vi "Start FTE Command.vi"(8 "error in":errorcluster, 10 "Start FTE":i64, 11 "CIFCorePlugin in":refnum<class "CIFCorePlugin.lvclass">) -> (0 "error out":errorcluster, 3 "CIFCorePlugin out":refnum<class "CIFCorePlugin.lvclass">)   [LabVIEW 2021, in "CIFCorePlugin.lvclass"]
uses:
  CIFCorePlugin.lvclass
  CIFCorePlugin.lvclass/CIFCorePlugin.ctl
  Typedef/gRPC to Main Command Payload.ctl
  Typedef/gRPC to Main Commands.ctl
  50968075-8c01-466c-b517-9351d77275d7.vi
  <vilib>/CIF Foundation/CIF CIPC/SubVIs/Check Error.vi
  <vilib>/CIF Foundation/CIF CIPC/SubVIs/Notify Of New Write.vi
  <vilib>/CIF Foundation/CIF CIPC/SubVIs/Get dll Path.vi
  <vilib>/CIF Foundation/CIF CIPC/SubVIs/Get Element Write Position.vi
  <vilib>/CIF Foundation/CIF CIPC/SubVIs/Get Element Info Variant.vi
  <vilib>/Utility/error.llb/Trim Whitespace.vi
  <vilib>/Utility/error.llb/Error Cluster From Error Code.vi
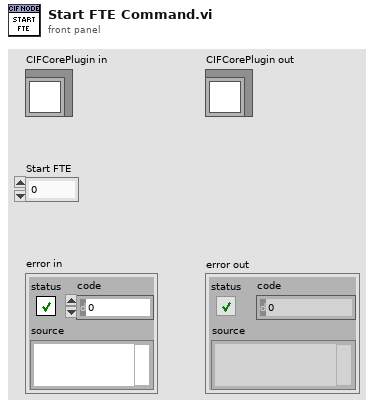
[diagram p1: front panel]
types:
  T1 = typedef "CIFCorePlugin.lvclass/gRPC to Main Command Payload.ctl" = cluster{"OOB_Rx Command":T2, "Array Index":i32}
  T2 = typedef "CIFCorePlugin.lvclass/gRPC to Main Commands.ctl" = enum8{"Start", "Pause", "Stop", "RefreshStats", "UpdateConfig", "Update Clock Map", "Connect Channel", "Force Channel", "Add Publisher Instance", "Remove Publisher Instance", "Prepare"}
  T3 = typedef "CIFCorePlugin.lvclass/gRPC to Main DVR.ctl" = refnum<data-value>
  T4 = typedef "CIFCoreCommon.lvlib/gRPC to Main Data.ctl" = cluster{"Config Data":variant, "Connections":T5[], "Forces":T6[], "Clock Conversion":T7, "Publisher Instance":T9, "Start FTE":i64}
  T5 = typedef "CIFCoreCommon.lvlib/Channel Connection Data.ctl" = cluster{"Publisher Name":string, "Subscriber Name":string, "Connection Data":u8[]}
  T6 = typedef "CIFCoreCommon.lvlib/Channel Force Data.ctl" = cluster{"Channel Name":string, "Force Data":u8[], "Force Active":bool}
  T7 = typedef "Time_CIF_U.lvlib/Clock Conversion Map.ctl" = map{u8, cluster{"Last Reset":i64, "Offset Pair":T8, "Slope":dbl, "1/Slope":dbl}}
  T8 = typedef "Time_CIF_U.lvlib/Timestamp Pair.ctl" = cluster{"System Time":i64, "External Time":i64}
  T9 = typedef "CIFCoreCommon.lvlib/FIFO Publisher.ctl" = cluster{"Publisher Name":string, "New FIFO Instance Config":T10}
  T10 = typedef "ChannelCommon.lvlib/New FIFO Instance Configuration.ctl" = cluster{"Backpressure":bool, "Bytes/Message Override":u32, "Messages/FIFO Override":u32, "Custom Data":u8[]}
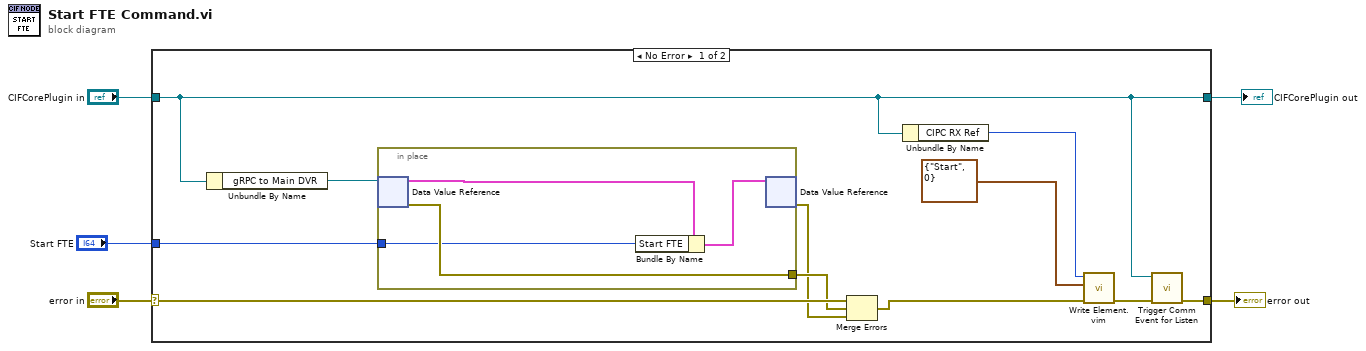
[diagram p0: block diagram]
diagram:
  n1 = case shown="No Error" "error in" {
    selector: "error in" -> [w14 w22]
    tunnel: [w7 w22] -> w2
    tunnel: "CIFCorePlugin in" -> [w6 w21]
    tunnel: [w6 w21] -> w3
    tunnel: "Start FTE" -> [w10 _]
    frame No Error {
      n2 = Unbundle By Name(w6) -> ("gRPC to Main DVR"=w15:T3)
      n3 = in-place {
        in-place-border: w10 -> [w17]
        in-place-border: [w19] -> w13
        n4 = in-place-dvr #1(w15) -> (w18:T4, w19:errorcluster)
        n5 = Bundle By Name(cluster=w18, "Start FTE"=w17) -> (w20:T4)
        n6 = in-place-dvr #1(w20) -> (w12:errorcluster)  [unwired: 1 out]
      }
      n7 = Merge Errors(w14, w13, w12) -> (w11:errorcluster)
      n8 = Unbundle By Name(w6) -> ("CIPC RX Ref"=w16:u64)
      n9 = call "Write Element.vim"("error in (no error)"=w11, "Data in"=T1 {"OOB_Rx Command"=enum."Start", "Array Index"=0} ("gRCP to Main Command Payload"), "CIPC Reference in"=w16) -> ("error out"=w8:errorcluster)  [unwired: 5 in, 3 out]
      n10 = call "Trigger Comm Event for Listen.vi"("error in (no error)"=w8, "CIFCorePlugin in"=w6) -> ("error out"=w7:errorcluster)  [unwired: 9 in]
    }
    frame Error {
    }
  }
  "error out" <- w2
  "CIFCorePlugin out" <- w3
